vi "DBInsertReadingVal.vi"(0 "db connection in":T1, 1 "sensor id":i32, 2 "timestamp":string, 3 "error in (no error)":errorcluster, 4 "reading value":dbl) -> (7 "db connection out":T1, 10 "error out":errorcluster)   [LabVIEW 2016]
uses:
  <vilib>/addons/database/Connection.llb/Conn ObjectReference.ctl
  Controls/DB Readings Columns.ctl
  Controls/DB Readings.ctl
  <vilib>/addons/database/NI_Database_API.lvlib
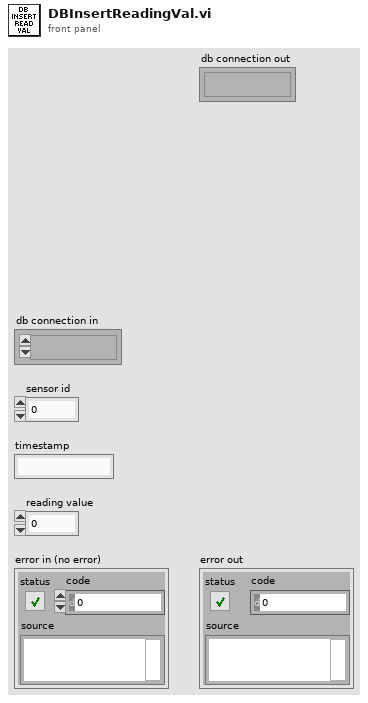
[diagram p1: front panel]
types:
  T1 = typedef "NI_Database_API.lvlib/Conn ObjectReference.ctl" = refnum<k1>
  T2 = typedef "DB Readings.ctl" = cluster{"reading_value":dbl, "sensor_id":i32, "reading_time":string}
  T3 = typedef "DB Readings Columns.ctl" = string[]
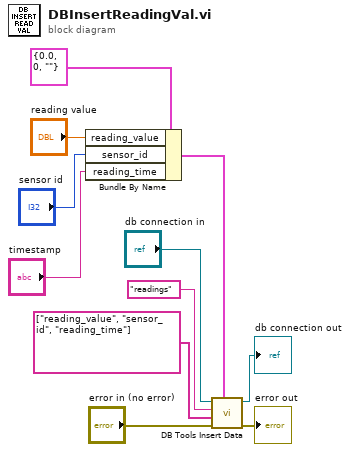
[diagram p0: block diagram]
diagram:
  n1 = Bundle By Name(cluster=T2 {"reading_value"=0.0, "sensor_id"=0, "reading_time"=""} ("readings cluster"), "reading_value"="reading value", "sensor_id"="sensor id", "reading_time"="timestamp") -> (w8:T2)
  n2 = call <vilib>:"DB Tools Insert Data.vi"("data"=w8, "error in (no error)"="error in (no error)", "columns"=T3 ["reading_value", "sensor_id", "reading_time"], "table"="readings", "connection reference"="db connection in") -> ("error out"=→"error out":errorcluster, "connection reference out"=→"db connection out":T1)  [unwired: 5 in]
